vi "lib Unix Time to Timestamp.vi"(8 "error in (no error)":errorcluster, 11 "unix timestamp":dbl) -> (0 "error out":errorcluster, 3 "time stamp":timestamp format="%<%H:%M:%S\n%x>T")   [LabVIEW 2016]
panel:
  in  "Unix Basetime":timestamp=timestamp(2082844800 s since 1904-01-01)
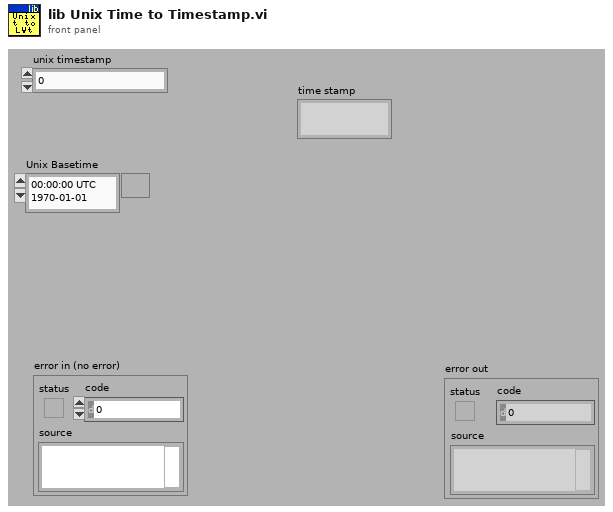
[diagram p1: front panel]
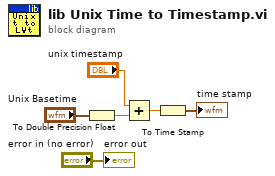
[diagram p0: block diagram]
diagram:
  n1 = To Double Precision Float(number="Unix Basetime") -> (double precision float=w5:dbl)
  n2 = Add(x="unix timestamp", y=w5) -> (x+y=w4:dbl)
  n3 = To Time Stamp(1:w4) -> (0:→"time stamp":timestamp)
  "error out" <- "error in (no error)"
